vi "All close.vi"(7 "Operation (Check)":enum16{"Init", "Check"}(ring)=enum."Check", 8 "Error In":errorcluster, 10 "Close? (F)":bool) -> (0 "Error Out":errorcluster, 2 "Close":bool)   [LabVIEW 2016]
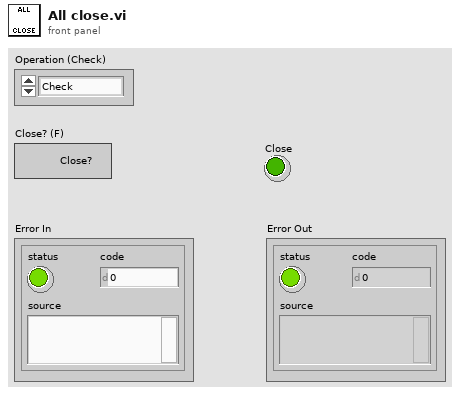
[diagram p1: front panel]
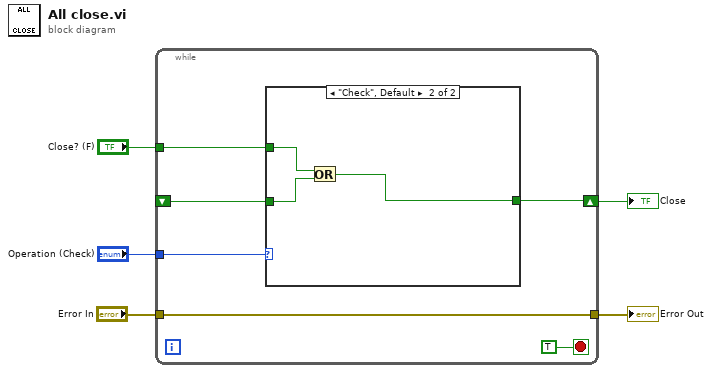
[diagram p0: block diagram]
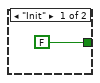
[diagram p2: hidden frame]
diagram:
  n1 = while {
    shift-right: [w9] -> w3
    shift-left: _ -> [w8]
    tunnel: "Close? (F)" -> [w7]
    tunnel: "Operation (Check)" -> [w10]
    tunnel: [w6] -> w1
    tunnel: "Error In" -> [w6]
    stop <- TRUE stop-if-true
    n2 = case shown="\"Check\", Default" w10 {
      tunnel: [FALSE w13] -> w9
      tunnel: w8 -> [_ w15]
      tunnel: w7 -> [_ w14]
      frame "Init" {
      }
      frame "Check", Default {
        n3 = Or(x=w14, y=w15) -> (x .or. y?=w13:bool)
      }
    }
  }
  "Close" <- w3
  "Error Out" <- w1
